vi "例6-17.vi"() -> ()   [LabVIEW 2019]
uses:
  <vilib>/Analysis/4window.llb/Hamming Window (DBL).vi
  <vilib>/Analysis/4window.llb/AllCosWindow (DBL).vi
  <vilib>/Analysis/NI_AALPro.lvlib
  <vilib>/Analysis/NI_AALBase.lvlib
panel:
  in  "采样点数":dbl=1000.0
  in  "采样频率":dbl=1000.0
  in  "信号相位":dbl=90.0
  in  "信号幅值":dbl=2.0
  in  "信号频率":dbl=10.57
  out "加窗后频谱":T1(graph)
  out "未加窗频谱":T1(graph)
  out "加窗后信号":cluster{i32, dbl, "Windowed X":dbl[]}(graph)
  out "原始信号":cluster{i32, dbl, "sine wave":dbl[]}(graph)
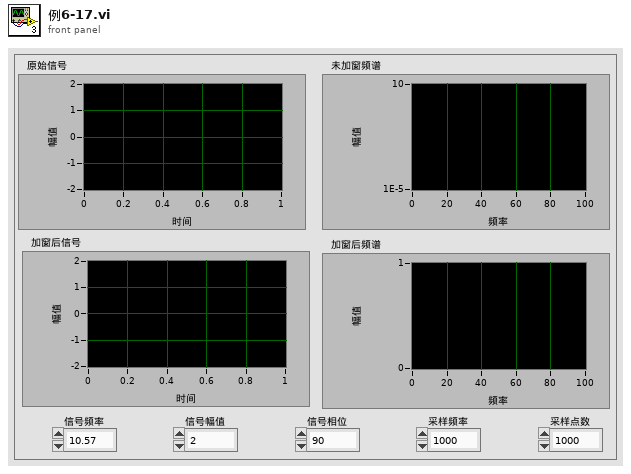
[diagram p1: front panel]
types:
  T1 = cluster{i32, "df":dbl, "Power Spectrum (V^2 rms)":dbl[]}
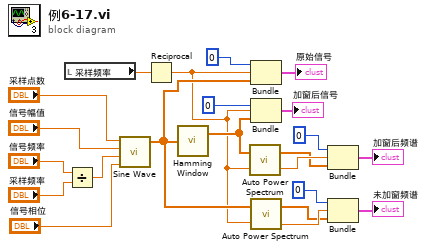
[diagram p0: block diagram]
diagram:
  n1 = local read "采样频率"() -> (w15:dbl)
  n2 = Divide(x="信号频率", y="采样频率") -> (x/y=w18:dbl)
  n3 = call <vilib>:"Sine Wave.vi"("samples"="采样点数", "amplitude"="信号幅值", "frequency"=w18, "phase in"="信号相位") -> ("sine wave"=w2:dbl[])  [unwired: 1 in, 2 out]
  n4 = Reciprocal(x=w15) -> (1/x=w1:dbl)
  n5 = call-poly <vilib>:"Hamming Window.vi"("X"=w2) -> ("Windowed X"=w12:dbl[])  [unwired: 1 out]
  n6 = call <vilib>:"Auto Power Spectrum.vi"("dt"=w1, "Signal (V)"=w12) -> ("df"=w8:dbl, "Power Spectrum (V^2 rms)"=w7:dbl[])
  n7 = Bundle(0, w1, "sine wave"=w2) -> (→"原始信号":cluster{i32, dbl, "sine wave":dbl[]})  [unwired: 1 in]
  n8 = Bundle(0, w1, "Windowed X"=w12) -> (→"加窗后信号":cluster{i32, dbl, "Windowed X":dbl[]})  [unwired: 1 in]
  n9 = call <vilib>:"Auto Power Spectrum.vi"("dt"=w1, "Signal (V)"=w2) -> ("df"=w6:dbl, "Power Spectrum (V^2 rms)"=w5:dbl[])
  n10 = Bundle(0, "df"=w8, "Power Spectrum (V^2 rms)"=w7) -> (→"加窗后频谱":T1)  [unwired: 1 in]
  n11 = Bundle(0, "df"=w6, "Power Spectrum (V^2 rms)"=w5) -> (→"未加窗频谱":T1)  [unwired: 1 in]
